vi "Run_Core.vi"(0 "Message Popup in":refnum<class "Generate Random Data.lvclass">, 11 "error in (no error)":errorcluster) -> (4 "Message Popup out":refnum<class "Generate Random Data.lvclass">, 6 "Return":variant, 15 "error out":errorcluster)   [LabVIEW 2016, in "Generate Random Data.lvclass"]
uses:
  Generate Random Data.lvclass
  E:/Repository/LabVIEW Script Language/source code/LSL components/functions/functionsbase/functionbase.lvclass
  functionsbase/functionbase.lvclass/functionbase.ctl
  functionsbase/properties/Read Smart Syntax Representation.vi
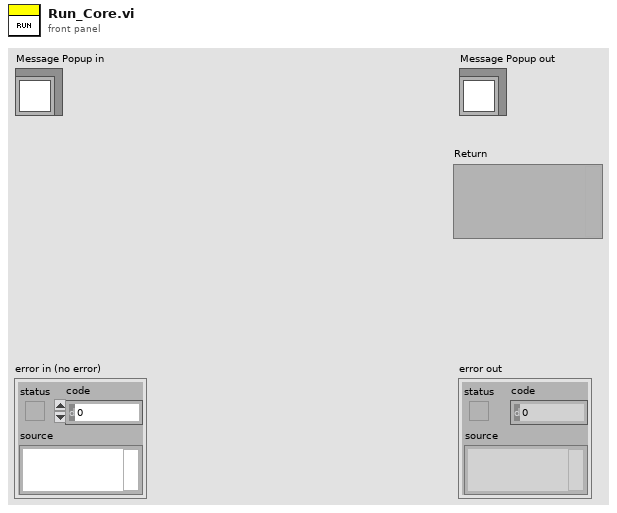
[diagram p1: front panel]
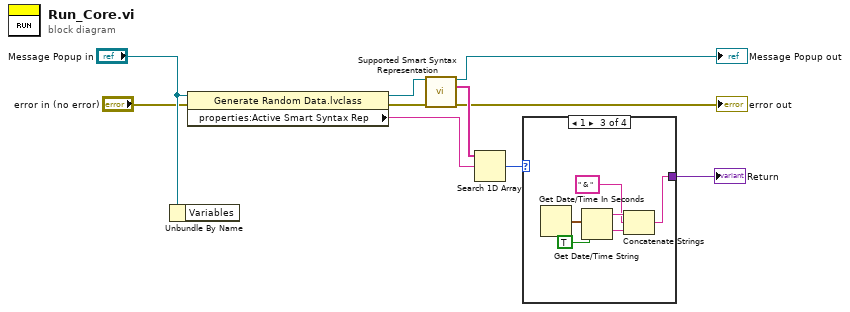
[diagram p0: block diagram]
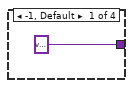
[diagram p2: hidden frame]
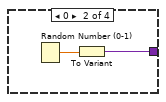
[diagram p3: hidden frame]
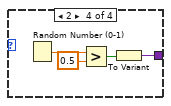
[diagram p4: hidden frame]
diagram:
  n1 = Unbundle By Name("Message Popup in") -> ()  [unwired: 1 out]
  n2 = property class="Generate Random Data.lvclass"(reference="Message Popup in", error in="error in (no error)") -> (reference out=w9:refnum<class "Generate Random Data.lvclass">, error out=w10:errorcluster, "properties:Active Smart Syntax Rep"=w4:string)
  n3 = call-dynamic "Supported Smart Syntax Representation.vi"("Message Popup in"=w9, "error in (no error)"=w10) -> ("Message Popup out"=→"Message Popup out":refnum<class "Generate Random Data.lvclass">, "Smart Syntax Representation List"=w5:string[], "error out"=→"error out":errorcluster)  [unwired: 11 in]
  n4 = Search 1D Array(1D array=w5, element=w4) -> (index of element=w2:i32)  [unwired: 1 in]
  n5 = case shown="1" w2 {
    tunnel: [variant ("Variant") w12 w16 w20] -> w1
    frame -1, Default {
    }
    frame 0 {
      n6 = Random Number (0-1)() -> (number: 0 to 1=w13:dbl)
      n7 = To Variant(anything=w13) -> (Variant=w12:variant)
    }
    frame 1 {
      n8 = Get Date/Time In Seconds() -> (seconds since 1Jan1904=w19:timestamp)
      n9 = Get Date/Time String(seconds (now)=w19, want seconds? (F)=TRUE) -> (date string=w18:string, time string=w17:string)  [unwired: 1 in]
      n10 = Concatenate Strings(w18, " & " ("string"), w17) -> (w16:string)
    }
    frame 2 {
      n11 = Random Number (0-1)() -> (number: 0 to 1=w23:dbl)
      n12 = Greater?(x=w23, y=0.5) -> (0:w21:bool)
      n13 = To Variant(anything=w21) -> (Variant=w20:variant)
    }
  }
  "Return" <- w1
